vi "getCategoryUpdateQuery.vi"(8 "error in (no error)":errorcluster, 10 "Name":string, 11 "Transaction in":refnum<class "Transaction.lvclass">) -> (0 "error out":errorcluster, 2 "Update Query":string, 3 "Transaction out":refnum<class "Transaction.lvclass">)   [LabVIEW 2018, in "Transaction.lvclass"]
uses:
  Transaction.lvclass
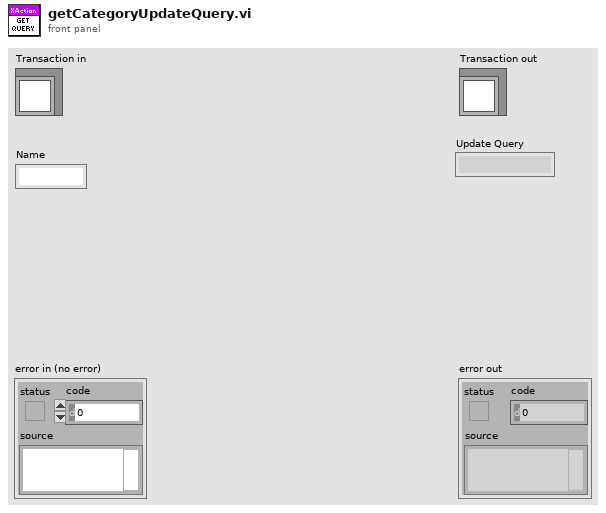
[diagram p1: front panel]
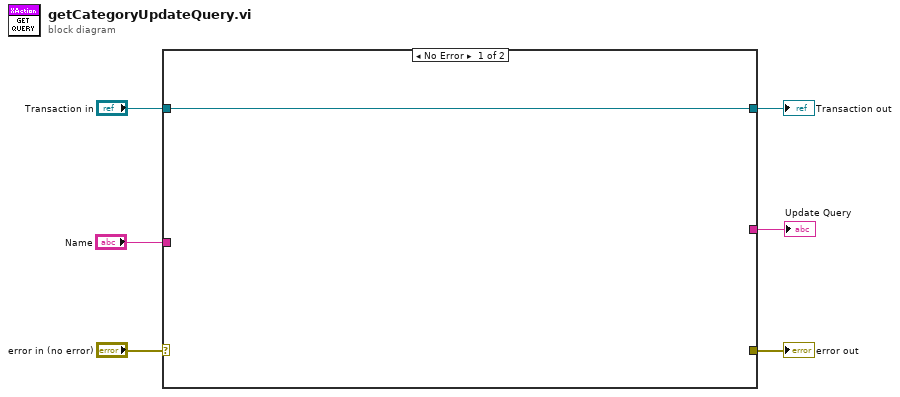
[diagram p0: block diagram]
diagram:
  n1 = case shown="No Error" "error in (no error)" {
    selector: "error in (no error)" -> [w9 w11]
    tunnel: [w8 w11] -> w5
    tunnel: [w7 w10] -> w3
    tunnel: "Transaction in" -> [w7 w10]
    tunnel: "Name" -> [_ _]
    tunnel: [_ _] -> w1
    frame No Error {
    }
    frame Error {
    }
  }
  "error out" <- w5
  "Transaction out" <- w3
  "Update Query" <- w1
